vi "OffsetMultiplier.vi"(0 "Array":dbl[](array[numeric])) -> (1 "Offset":dbl, 2 "Multiplier":dbl)   [LabVIEW 2016]
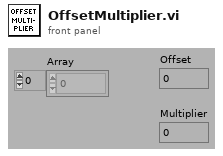
[diagram p1: front panel]
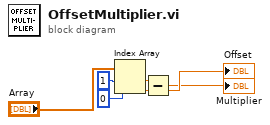
[diagram p0: block diagram]
diagram:
  n1 = Index Array(array="Array", index #1=1 ("index"), index #2=0 ("index")) -> (element #1=w3:dbl, element #2=w6:dbl)
  "Offset" <- w6
  n2 = Subtract(x=w3, y=w6) -> (x-y=→"Multiplier":dbl)
